vi "test.vi"() -> ()   [LabVIEW 2014]
panel:
  out "Boolean":bool
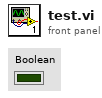
[diagram p1: front panel]
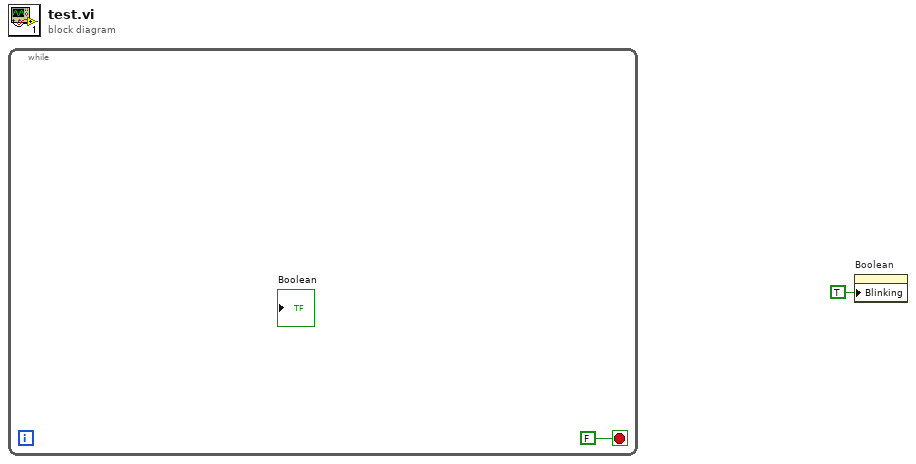
[diagram p0: block diagram]
diagram:
  n1 = while {
    stop <- FALSE stop-if-true
  }
  n2 = property on="Boolean" class="Bool (strict)"("Blinking"=TRUE) -> ()  [unwired: 2 in, 2 out]
